vi "ReadRCMFileToRCMDatum.vi"(8 "error in (no error)":errorcluster, 10 "item name (\"\": root)":string, 11 "rcm file path":path) -> (0 "error out":errorcluster, 3 "rcm datum":T1[](array[typedef]))   [LabVIEW 2009]
uses:
  Type Definitions/RCMData.ctl
  Support/MSXML/Public/Type Definition/Attribute__slk_msxml.ctl
  Support/MSXML/Public/MSXML Document/msxml document.lvclass
  Support/MSXML/Public/MSXML Node/msxml node.lvclass
  Support/MSXML/Library/MSXML.lvlib
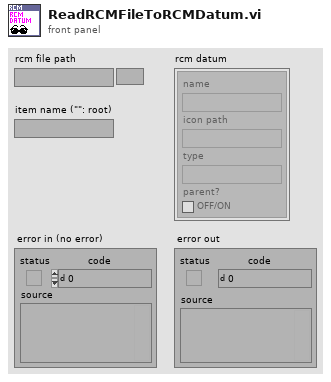
[diagram p1: front panel]
types:
  T1 = typedef "RCMData.ctl" = cluster{"name":string, "icon path":path, "type":string, "parent?":bool}
  T2 = typedef "MSXML.lvlib/Attribute__slk_msxml.ctl" = cluster{"name":string, "value":string}
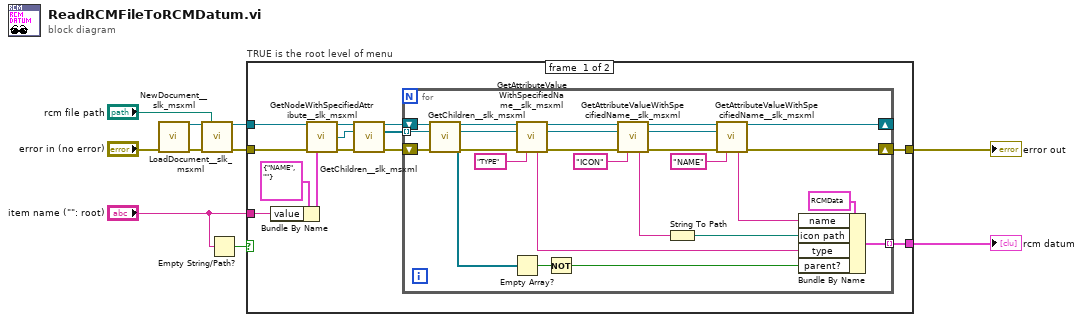
[diagram p0: block diagram]
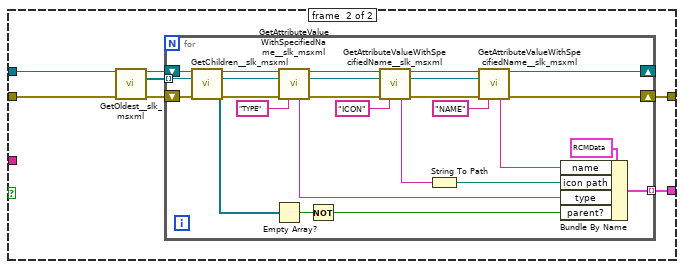
[diagram p2: hidden frame]
diagram:
  n1 = call "NewDocument__slk_msxml.vi"("error in (no error)"="error in (no error)") -> ("document out"=w10:refnum<class "msxml document.lvclass">, "error out"=w9:errorcluster)  [unwired: 13 in]
  n2 = call "LoadDocument__slk_msxml.vi"("document in"=w10, "xml document path in"="rcm file path", "error in (no error)"=w9) -> ("document out"=w5:refnum<class "msxml document.lvclass">, "error out"=w6:errorcluster)  [unwired: 11 in]
  n3 = Empty String/Path?(string/path="item name (\"\": root)") -> (empty?=w7:bool)
  n4 = case "TRUE is the root level of menu" shown="True" w7 {
    tunnel: w6 -> [w18 w50]
    tunnel: w5 -> [w23 w49]
    tunnel: "item name (\"\": root)" -> [w13 _]
    tunnel: [w12 w52] -> w3
    tunnel: [w11 w51] -> w2
    frame #0 {
      n5 = Bundle By Name(cluster=T2 {"name"="NAME", "value"=""} ("attribute"), "value"=w13) -> (w14:T2)
      n6 = call "GetNodeWithSpecifiedAttribute__slk_msxml.vi"("document in"=w23, "error in (no error)"=w18, "attribute"=w14) -> ("document out"=w19:refnum<class "msxml document.lvclass">, "first node out"=w16:refnum<class "msxml node.lvclass">, "error out"=w17:errorcluster)  [unwired: 9 in, 1 out]
      n7 = call "GetChildren__slk_msxml.vi"("document in"=w19, "parent node in"=w16, "error in (no error)"=w17) -> ("document out"=w22:refnum<class "msxml document.lvclass">, "children nodes out"=w20:refnum<class "msxml node.lvclass">[], "error out"=w21:errorcluster)  [unwired: 9 in, 1 out]
      n8 = for {
        shift-right: [w25] -> _
        shift-left: w22 -> [w43]
        shift-right: [w24] -> w11
        shift-left: w21 -> [w41]
        tunnel: w20 -> [w39] mode=indexing
        tunnel: [w47] -> w12 mode=indexing
        n9 = call "GetChildren__slk_msxml.vi"("document in"=w43, "parent node in"=w39, "error in (no error)"=w41) -> ("document out"=w42:refnum<class "msxml document.lvclass">, "children nodes out"=w38:refnum<class "msxml node.lvclass">[], "error out"=w40:errorcluster)  [unwired: 9 in, 1 out]
        n10 = Empty Array?(array=w38) -> (empty?=w37:bool)
        n11 = call "GetAttributeValueWithSpecifiedName__slk_msxml.vi"("document in"=w42, "node in"=w39, "error in (no error)"=w40, "attribute name"="TYPE") -> ("document out"=w28:refnum<class "msxml document.lvclass">, "node out"=w31:refnum<class "msxml node.lvclass">, "attribute value"=w35:string, "error out"=w29:errorcluster)  [unwired: 8 in]
        n12 = Not(x=w37) -> (.not. x?=w36:bool)
        n13 = call "GetAttributeValueWithSpecifiedName__slk_msxml.vi"("document in"=w28, "node in"=w31, "error in (no error)"=w29, "attribute name"="ICON") -> ("document out"=w27:refnum<class "msxml document.lvclass">, "node out"=w30:refnum<class "msxml node.lvclass">, "attribute value"=w33:string, "error out"=w26:errorcluster)  [unwired: 8 in]
        n14 = String To Path(string=w33) -> (path=w32:path)
        n15 = call "GetAttributeValueWithSpecifiedName__slk_msxml.vi"("document in"=w27, "node in"=w30, "error in (no error)"=w26, "attribute name"="NAME") -> ("document out"=w25:refnum<class "msxml document.lvclass">, "attribute value"=w34:string, "error out"=w24:errorcluster)  [unwired: 8 in, 1 out]
        n16 = Bundle By Name(cluster=T1 {"name"="", "icon path"=path "", "type"="", "parent?"=FALSE} ("rcm item data"), "name"=w34, "icon path"=w32, "type"=w35, "parent?"=w36) -> (w47:T1)
      }
    }
    frame #1 {
      n17 = call "GetOldest__slk_msxml.vi"("document in"=w49, "error in (no error)"=w50) -> ("document out"=w55:refnum<class "msxml document.lvclass">, "oldest nodes out"=w53:refnum<class "msxml node.lvclass">[], "error out"=w54:errorcluster)  [unwired: 10 in, 1 out]
      n18 = for {
        shift-right: [w59] -> _
        shift-left: w55 -> [w75]
        shift-right: [w58] -> w51
        shift-left: w54 -> [w73]
        tunnel: w53 -> [w71] mode=indexing
        tunnel: [w79] -> w52 mode=indexing
        n19 = call "GetChildren__slk_msxml.vi"("document in"=w75, "parent node in"=w71, "error in (no error)"=w73) -> ("document out"=w74:refnum<class "msxml document.lvclass">, "children nodes out"=w70:refnum<class "msxml node.lvclass">[], "error out"=w72:errorcluster)  [unwired: 9 in, 1 out]
        n20 = Empty Array?(array=w70) -> (empty?=w69:bool)
        n21 = call "GetAttributeValueWithSpecifiedName__slk_msxml.vi"("document in"=w74, "node in"=w71, "error in (no error)"=w72, "attribute name"="TYPE") -> ("document out"=w56:refnum<class "msxml document.lvclass">, "node out"=w63:refnum<class "msxml node.lvclass">, "attribute value"=w67:string, "error out"=w61:errorcluster)  [unwired: 8 in]
        n22 = Not(x=w69) -> (.not. x?=w68:bool)
        n23 = call "GetAttributeValueWithSpecifiedName__slk_msxml.vi"("document in"=w56, "node in"=w63, "error in (no error)"=w61, "attribute name"="ICON") -> ("document out"=w60:refnum<class "msxml document.lvclass">, "node out"=w62:refnum<class "msxml node.lvclass">, "attribute value"=w65:string, "error out"=w57:errorcluster)  [unwired: 8 in]
        n24 = String To Path(string=w65) -> (path=w64:path)
        n25 = call "GetAttributeValueWithSpecifiedName__slk_msxml.vi"("document in"=w60, "node in"=w62, "error in (no error)"=w57, "attribute name"="NAME") -> ("document out"=w59:refnum<class "msxml document.lvclass">, "attribute value"=w66:string, "error out"=w58:errorcluster)  [unwired: 8 in, 1 out]
        n26 = Bundle By Name(cluster=T1 {"name"="", "icon path"=path "", "type"="", "parent?"=FALSE} ("rcm item data"), "name"=w66, "icon path"=w64, "type"=w67, "parent?"=w68) -> (w79:T1)
      }
    }
  }
  "rcm datum" <- w3
  "error out" <- w2
